vi "Is Big Endian.vi"() -> (0 "big endian":bool)   [LabVIEW 2017, in "Palette Menu.lvlib" / "ResMgr.lvlib"]
uses:
  <vilib>/Palette API/ResMgr/ResMgr.lvlib
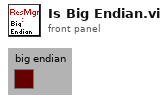
[diagram p1: front panel]
types:
  T1 = enum16{"big-endian, network order", "native, host order", "little-endian"}
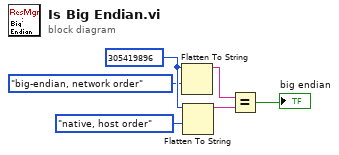
[diagram p0: block diagram]
diagram:
  w6 = 305419896 ("Input Value")
  n1 = Flatten To String(anything=w6, byte order (0:big-endian, network order)=T1."big-endian, network order") -> (data string=w3:string)  [unwired: 1 in, 3 out]
  n2 = Flatten To String(anything=w6, byte order (0:big-endian, network order)=T1."native, host order") -> (data string=w2:string)  [unwired: 1 in, 3 out]
  n3 = Equal?(x=w3, y=w2) -> (x = y?=→"big endian":bool)
